vi "Temp_Control_V_Peltier control example PID.vi"() -> ()   [LabVIEW 2013]
uses:
  <vilib>/Analysis/baseanly.llb/Mean (DBL).vi
  <vilib>/Analysis/NI_AALBase.lvlib
panel:
  in  "Current":dbl(slide) scale=0.0..1.0
  in  "Stop (Esc)":bool
  out "Temperature":dbl[](graph)
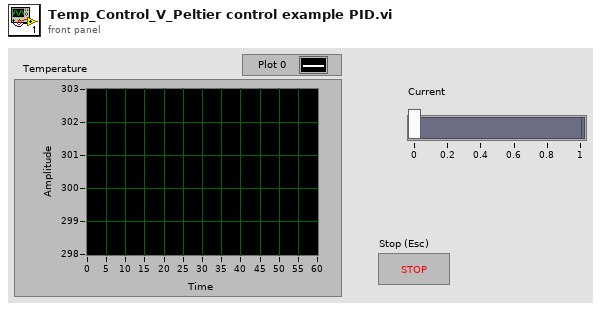
[diagram p1: front panel]
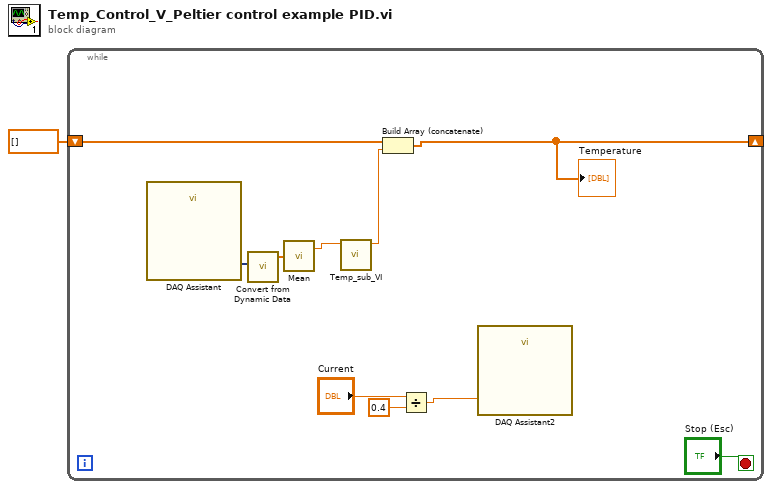
[diagram p0: block diagram]
diagram:
  n1 = while {
    shift-right: [w6] -> _
    shift-left: dbl[] [] -> [w7]
    stop <- "Stop (Esc)" stop-if-true
    n2 = call "DAQ Assistant"() -> ("data"=w11:dynamicdata)  [unwired: 17 in, 2 out]
    n3 = call "Convert from Dynamic Data"("Dynamic Data Type"=w11) -> ("Array"=w10:dbl[])  [unwired: 3 in]
    n4 = call-poly <vilib>:"Mean.vi"("X"=w10) -> ("mean"=w9:dbl)  [unwired: 1 out]
    n5 = call "Temp_sub_VI.vi"("mean"=w9) -> ("T"=w8:dbl)  [unwired: 10 in]
    n6 = Build Array (concatenate)(w7, w8) -> (w6:dbl[])
    "Temperature" <- w6
    n7 = Divide(x="Current", y=0.4) -> (x/y=w2:dbl)
    n8 = call "DAQ Assistant2"("data"=w2) -> ()  [unwired: 17 in, 2 out]
  }
